vi "Disconnect.vi"(8 "error in":errorcluster, 11 "69X_79X in":refnum<class "69X_79X.lvclass">) -> (0 "error out":errorcluster, 3 "69X_79X out":refnum<class "69X_79X.lvclass">)   [LabVIEW 2019, in "69X_79X.lvlib" / "69X_79X.lvclass"]
uses:
  Library/69X_79X.lvclass
  Library/69X_79X.lvclass/69X_79X.ctl
  <instrlib>/Agilent N6900 N7900 Series/Agilent N6900 N7900 Series.lvlib
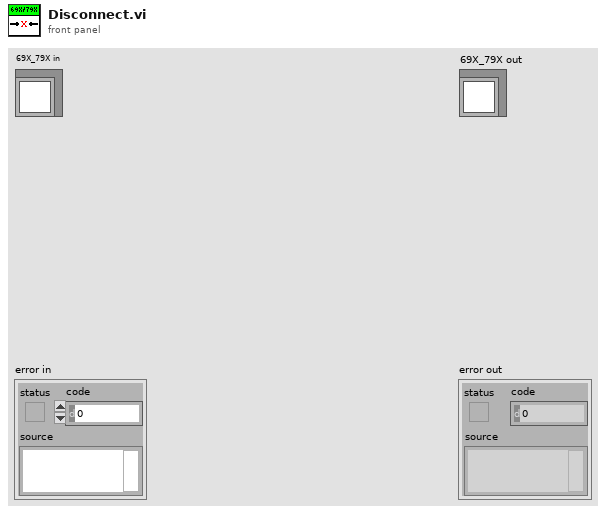
[diagram p1: front panel]
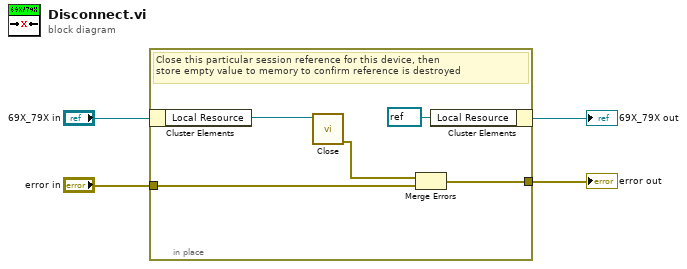
[diagram p0: block diagram]
diagram:
  n1 = in-place {
    in-place-border: "error in" -> [w8]
    in-place-border: [w6] -> w2
    # "Close this particular session reference for this device, then\nstore empty value to memory to confirm reference is destroyed"
    n2 = in-place-cluster #1("69X_79X in") -> ("Local Resource"=w9:refnum<visa-resource-name>)
    n3 = call <instrlib>:"Close.vi"("VISA resource name"=w9) -> ("error out"=w7:errorcluster)  [unwired: 10 in]
    n4 = Merge Errors(w7, w8) -> (w6:errorcluster)
    n5 = in-place-cluster #1("Local Resource"=refnum<visa-resource-name> refnum) -> (→"69X_79X out":refnum<class "69X_79X.lvclass">)
  }
  "error out" <- w2
